vi "MotionProfileControlsInit.vi"   [LabVIEW 2017]
uses:
  General/MotionProfiling/TypeDefs/TrajectoryPoint.ctl
  <vilib>/Rock Robotics/WPI/ThirdParty/Phoenix-LabVIEW/Motor Controller/Controls/CTRE_Phoenix_MotorControl_TrajectoryPointTimeDur.ctl
  General/MotionProfiling/TypeDefs/MotionProfileControl.ctl
  MotionProfileControlData.vi
types:
  T1 = typedef "MotionProfileControl.ctl" = cluster{"ControlMutex":T2, "Trajectory Points":T3[], "CurrentIndex":u32}
  T2 = typedef "Semaphore RefNum" = refnum<k1>
  T3 = typedef "TrajectoryPoint.ctl" = cluster{"Position ":dbl, "Velocity ":dbl, "Time (ms)":T4, "Last Point":bool}
  T4 = typedef "CTRE_Phoenix_MotorControl_TrajectoryPointTimeDur.ctl" = i32
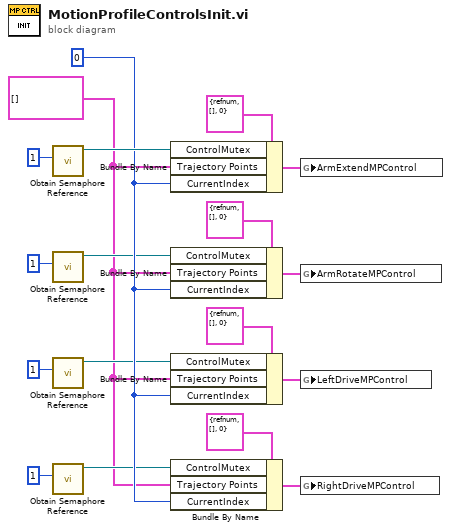
[diagram p0: block diagram]
diagram:
  w5 = u32 0 ("ArmExtendMPControl.CurrentIndex")
  w1 = T3[] [] ("ArmExtendMPControl.Trajectory Points")
  n1 = call <vilib>:"Obtain Semaphore Reference.vi"("size (1)"=1) -> ("semaphore"=w18:T2)  [unwired: 4 in, 2 out]
  n2 = call <vilib>:"Obtain Semaphore Reference.vi"("size (1)"=1) -> ("semaphore"=w4:T2)  [unwired: 4 in, 2 out]
  n3 = call <vilib>:"Obtain Semaphore Reference.vi"("size (1)"=1) -> ("semaphore"=w3:T2)  [unwired: 4 in, 2 out]
  n4 = call <vilib>:"Obtain Semaphore Reference.vi"("size (1)"=1) -> ("semaphore"=w2:T2)  [unwired: 4 in, 2 out]
  n5 = Bundle By Name(cluster=T1 {"ControlMutex"=refnum, "Trajectory Points"=[], "CurrentIndex"=0} ("MotionProfileControl"), "ControlMutex"=w18, "Trajectory Points"=w1, "CurrentIndex"=w5) -> (w13:T1)
  n6 = Bundle By Name(cluster=T1 {"ControlMutex"=refnum, "Trajectory Points"=[], "CurrentIndex"=0} ("MotionProfileControl"), "ControlMutex"=w4, "Trajectory Points"=w1, "CurrentIndex"=w5) -> (w10:T1)
  n7 = Bundle By Name(cluster=T1 {"ControlMutex"=refnum, "Trajectory Points"=[], "CurrentIndex"=0} ("MotionProfileControl"), "ControlMutex"=w3, "Trajectory Points"=w1, "CurrentIndex"=w5) -> (w9:T1)
  n8 = Bundle By Name(cluster=T1 {"ControlMutex"=refnum, "Trajectory Points"=[], "CurrentIndex"=0} ("MotionProfileControl"), "ControlMutex"=w2, "Trajectory Points"=w1, "CurrentIndex"=w5) -> (w6:T1)
  n9 = global write "MotionProfileControlData.vi" "ArmExtendMPControl"(w13) -> ()
  n10 = global write "MotionProfileControlData.vi" "ArmRotateMPControl"(w10) -> ()
  n11 = global write "MotionProfileControlData.vi" "LeftDriveMPControl"(w9) -> ()
  n12 = global write "MotionProfileControlData.vi" "RightDriveMPControl"(w6) -> ()
